vi "Main.vi"(8 "error in":errorcluster, 11 "data server thread in":refnum<class "Data Server Thread.lvclass">) -> (0 "error out":errorcluster, 3 "data server thread out":refnum<class "Data Server Thread.lvclass">)   [LabVIEW 2021, in "DSF Core.lvlib" / "Data Server Thread.lvclass"]
uses:
  Data Server Thread.lvclass
  C:/dev/git/custom-devices/niveristand-data-sharing-framework-custom-device/Source/Core/Classes/Thread/Thread.lvclass
  Data Server Thread.lvclass/Data Server Thread.ctl
  Transfer/Transfer.lvclass/Transfer.ctl
  Buffers/Buffers.lvclass/Buffers.ctl
  <vilib>/NI/Memory Manager/Classes/Pointer/Pointer.lvclass/Pointer.ctl
  Thread.lvclass/Thread.ctl
  <vilib>/NI/Memory Manager/Classes/Pointer/Read.vi
  <vilib>/NI/Memory Manager/Classes/Pointer/Read Bool.vi
  Serve Configuration.vi
  Serve Buffer to Connection.vi
  Status/Read Status.vi
  Check for Buffer Request.vi
  Get Transfer Buffers.vi
  Remove Viewer.vi
  <vilib>/NI/Memory Manager/Classes/Pointer/Read (No Check).vi
  <vilib>/NI/Memory Manager/Classes/Pointer/Read (No Check) Bool.vi
  <vilib>/NI/Memory Manager/Classes/Pointer/Check Move.vi
  <vilib>/NI/Memory Manager/Classes/Pointer/Is Null.vi
  Buffer/Get Buffer Size.vi
  Buffer/Read Buffer 1D U8.vi
  <vilib>/NI/Memory Manager/Classes/Pointer/Check Size.vi
  <vilib>/NI/Memory Manager/Classes/Pointer/Get Address.vi
  Status/Status Size.vi
  <vilib>/NI/Memory Manager/Classes/Pointer/Check Null Pointer.vi
  Transfer/Get Transfer Buffers.vi
  <vilib>/NI/Memory Manager/Classes/Pointer/Subset.vi
  <vilib>/NI/Memory Manager/Classes/Pointer/Check Count.vi
  <vilib>/NI/Memory Manager/Classes/Pointer/Check Bounds (Power of 2).vi
  <vilib>/NI/Memory Manager/Classes/Pointer/Get Size.vi
  <vilib>/NI/Memory Manager/Classes/Pointer/Read 1D U8.vi
  <vilib>/NI/Memory Manager/Classes/Pointer/Errors.vi
  <vilib>/NI/Memory Manager/Classes/Pointer/Out of Bounds.vi
  <vilib>/NI/Memory Manager/Classes/Pointer/Null Pointer.vi
  Buffers/Get Active Buffers.vi
  <vilib>/NI/Memory Manager/Classes/Pointer/Encapsulate.vi
  <vilib>/NI/Memory Manager/Classes/Pointer/Check Length.vi
  <vilib>/NI/Memory Manager/Classes/Pointer/Check Bounds.vi
  <vilib>/NI/Memory Manager/Classes/Pointer/Read (No Check) 1D U8.vi
  <vilib>/NI/Memory Manager/VIs/Write String to Source.vi
  <vilib>/NI/Memory Manager/Classes/Pointer/Write Pointer Size to Error.vi
  <vilib>/NI/Memory Manager/Classes/Pointer/Create Error.vi
  <vilib>/NI/Memory Manager/VIs/Write Numeric to Source.vi
  <vilib>/NI/Memory Manager/VIs/Write Numeric Scalar to Source (Base10 U64).vi
  <vilib>/NI/Memory Manager/Classes/Pointer/Set Size.vi
  <vilib>/NI/Memory Manager/Classes/Pointer/Set Address.vi
  <vilib>/NI/Memory Manager/Classes/Pointer/Set Internal.vi
  <vilib>/NI/Memory Manager/Classes/Pointer/Check Bounds (Pointer).vi
  <vilib>/NI/Memory Manager/Classes/Pointer/Check Bounds (Buffer).vi
  <vilib>/NI/Memory Manager/VIs/New Error Cluster.vi
  <vilib>/NI/Memory Manager/VIs/New Error Cluster (512B).vi
  <vilib>/NI/Memory Manager/VIs/Set Error Status.vi
  <vilib>/NI/Memory Manager/VIs/Set Error Code.vi
  <vilib>/NI/Memory Manager/VIs/Set Error Source.vi
  <vilib>/NI/Memory Manager/Constants/Constants.vi
  <vilib>/NI/Memory Manager/Constants/Library Name.vi
  <vilib>/NI/Memory Manager/Classes/Pointer/Pointer Error Info.vi
  <vilib>/NI/Memory Manager/Constants/Pointer Class Name.vi
  <vilib>/NI/Memory Manager/Classes/Pointer/Buffer Underflow.vi
  Buffer/Buffer.lvclass
  C:/Program Files/National Instruments/LabVIEW 2021/vi.lib/NI/Memory Manager/Classes/Pointer/Pointer.lvclass
  Status/Status Pointer.lvclass
  Thread.lvclass
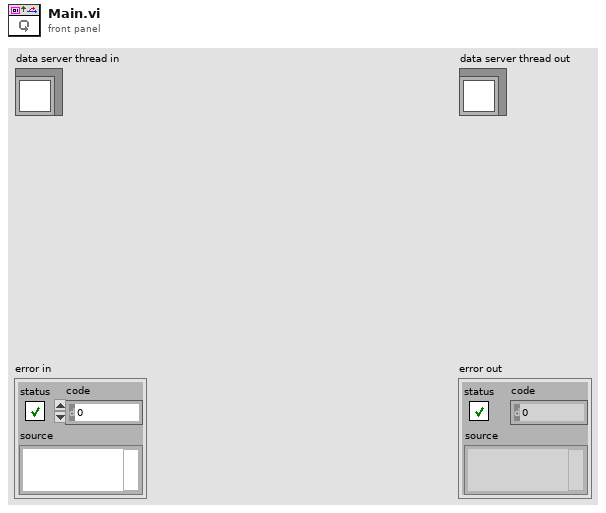
[diagram p1: front panel]
types:
  T1 = typedef "DSF Core.lvlib/Data Server Thread.lvclass/Viewer Data.ctl" = cluster{"remote address":string, "remote port":u16, "connection ID":refnum<k5>, "Buffer":refnum<class "Buffer.lvclass">, "Status":refnum<class "Status Pointer.lvclass">}
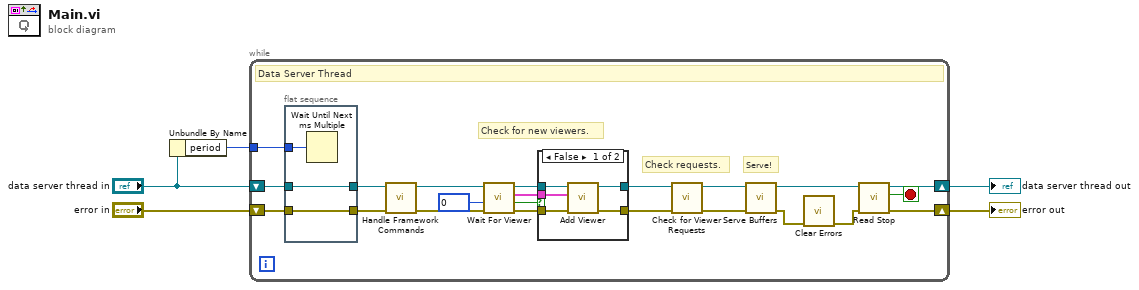
[diagram p0: block diagram]
diagram:
  n1 = Unbundle By Name("data server thread in") -> ("period"=w1:u32)
  n2 = while {
    shift-right: [w25] -> w5
    shift-left: "error in" -> [w18]
    shift-right: [w27] -> w4
    shift-left: "data server thread in" -> [w17]
    tunnel: w1 -> [w19]
    stop <- w26 stop-if-true
    # "Check requests."
    # "Serve!"
    # "Check for new viewers."
    # "Data Server Thread"
    n3 = flat-sequence {
      tunnel: w19 -> [w30]
      tunnel: w18 -> [w29]
      tunnel: w17 -> [w28]
      tunnel: [w29] -> w11
      tunnel: [w28] -> w12
      frame #0 {
        n4 = Wait Until Next ms Multiple(millisecond multiple=w30) -> ()  [unwired: 1 out]
      }
    }
    n5 = call "Handle Framework Commands.vi"("error in (no error)"=w11, "Data Server Thread in"=w12) -> ("error out"=w9:errorcluster, "Data Server Thread out"=w10:refnum<class "Data Server Thread.lvclass">)  [unwired: 8 in]
    n6 = call "Wait For Viewer.vi"("error in"=w9, "timeout ms (wait forever: -1)"=0, "Data Server Thread in"=w10) -> ("error out"=w21:errorcluster, "timed out?"=w23:bool, "viewer"=w20:T1, "Data Server Thread out"=w22:refnum<class "Data Server Thread.lvclass">)  [unwired: 5 in]
    n7 = case shown="False" w23 {
      tunnel: w22 -> [w35 w37]
      tunnel: w21 -> [w34 w36]
      tunnel: w20 -> [w33 _]
      tunnel: [w32 w36] -> w16
      tunnel: [w31 w37] -> w15
      frame False {
        n8 = call "Add Viewer.vi"("error in"=w34, "viewer"=w33, "Data Server Thread in"=w35) -> ("error out"=w32:errorcluster, "Data Server Thread out"=w31:refnum<class "Data Server Thread.lvclass">)  [unwired: 7 in]
      }
      frame True {
      }
    }
    n9 = call "Check for Viewer Requests.vi"("error in"=w16, "data server thread in"=w15) -> ("error out"=w14:errorcluster, "data server thread out"=w13:refnum<class "Data Server Thread.lvclass">)  [unwired: 8 in]
    n10 = call "Serve Buffers.vi"("error in"=w14, "data server thread in"=w13) -> ("error out"=w8:errorcluster, "data server thread out"=w7:refnum<class "Data Server Thread.lvclass">)  [unwired: 8 in]
    n11 = call <vilib>:"Clear Errors.vi"("error in (no error)"=w8) -> ("error out"=w6:errorcluster)  [unwired: 5 in, 1 out]
    n12 = call "Read Stop.vi"("error in (no error)"=w6, "Thread in"=w7) -> ("error out"=w25:errorcluster, "stop"=w26:bool, "Thread out"=w27:refnum<class "Data Server Thread.lvclass">)  [unwired: 7 in]
  }
  "error out" <- w5
  "data server thread out" <- w4
